vi "Ke2000 Measurement.vi"(7 "Source (0: Function)":u16(ring) items=["Function", "Calculation 1", "Calculation 2", "Calculation 3"], 8 "error in (no error)":errorcluster, 11 "VISA resource name":refnum<visa-resource-name>) -> (0 "error out":errorcluster, 1 "Units":string, 2 "Meas in micro":string, 3 "VISA resource name out":refnum<visa-resource-name>, 5 "Measurement":dbl, 10 "Channel":i32)   [LabVIEW 2012]
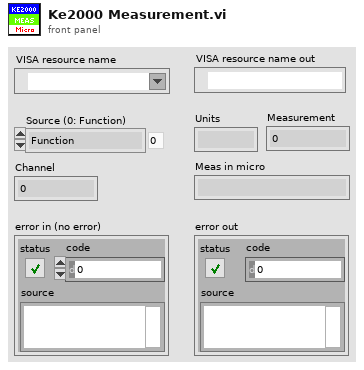
[diagram p1: front panel]
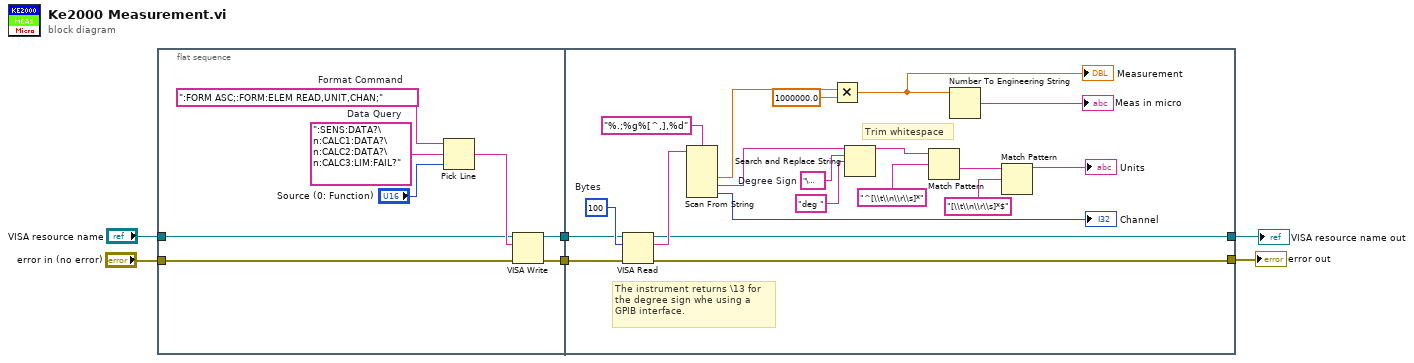
[diagram p0: block diagram]
diagram:
  n1 = flat-sequence {
    tunnel: "VISA resource name" -> [w8]
    tunnel: "error in (no error)" -> [w7]
    tunnel: [w11] -> w4
    tunnel: [w10] -> w3
    tunnel: w4 -> [w22]
    tunnel: w3 -> [w21]
    tunnel: [w20] -> w2
    tunnel: [w19] -> w1
    frame #0 {
      w13 = ":SENS:DATA?\n:CALC1:DATA?\n:CALC2:DATA?\n:CALC3:LIM:FAIL?"  # Data Query
      w14 = ":FORM ASC;:FORM:ELEM READ,UNIT,CHAN;"  # Format Command
      n2 = Pick Line(string ("")=w14, multi-line string=w13, line index="Source (0: Function)") -> (output string=w9:string)
      n3 = VISA Write(VISA resource name=w8, write buffer=w9, error in (no error)=w7) -> (VISA resource name out=w11:refnum<visa-resource-name>, error out=w10:errorcluster)  [unwired: 1 out]
    }
    frame #1 {
      w32 = "\u0013"  # Degree Sign
      w23 = u32 100  # Bytes
      # "Trim whitespace"
      # "The instrument returns \\13 for\nthe degree sign whe using a\nGPIB interface."
      n4 = VISA Read(VISA resource name=w22, byte count=w23, error in (no error)=w21) -> (VISA resource name out=w20:refnum<visa-resource-name>, read buffer=w34:string, error out=w19:errorcluster)  [unwired: 1 out]
      n5 = Scan From String(format string="%.;%g%[^,],%d", input string=w34) -> (output 1=w18:dbl, output 2=w31:string, output 3=→"Channel":i32)  [unwired: 5 in, 3 out]
      n6 = Multiply(x=w18, y=1000000.0) -> (x*y=w15:dbl)
      "Measurement" <- w15
      n7 = Search and Replace String(input string=w31, search string=w32, replace string="deg " ("replace string (\"\")")) -> (result string=w25:string)  [unwired: 5 in, 3 out]
      n8 = Match Pattern(string=w25, regular expression="^[\\t\\n\\r\\s]*") -> (after substring=w28:string)  [unwired: 1 in, 3 out]
      n9 = Number To Engineering String(4:w15) -> (0:→"Meas in micro":string)  [unwired: 3 in]
      n10 = Match Pattern(string=w28, regular expression="[\\t\\n\\r\\s]*$") -> (before substring=→"Units":string)  [unwired: 1 in, 3 out]
    }
  }
  "error out" <- w1
  "VISA resource name out" <- w2
